vi "Mcp2210 Write EE Prom.vi"(8 "error in (no error)":errorcluster, 9 "value":u8, 10 "address":u8, 11 "handle":i32) -> (0 "error out":errorcluster, 3 "handle out":i32)   [LabVIEW 2015, in "mcp2210.lvlib"]
doc: "Write one byte at the EEPROM memory address provided as parameter.\nThe EEPROM size is 256 bytes.\nThe function returns negative error code in case of failure.\nIf the error code is \"M_E_ERR_BLOCKED_ACCESS\" the write failure is due to the device being either\npassword protected or permanently locked. M_Mcp2210_GetAccessStatus() API provides the details about\ndevice protection status. If the device is not permanently locked, the password protection can be\nunlocked or disabled by using the access control API.\nParameters:\nInputs:\n- IntPtr handle - The USB device handle. Cannot be NULL.\n- unsigned char address - the EEPROM location to write to.\n- unsigned char content - the value to store at the EEPROM address.\nOutputs:\n- none\nReturns:\n- 0 for success: M_E_SUCCESS\n- negative error code: M_E_ERR_NULL, M_E_ERR_INVALID_HANDLE_VALUE\nM_E_ERR_HID_TIMEOUT, M_E_ERR_HID_RW_FILEIO, M_E_ERR_UNKOWN_ERROR\nM_E_ERR_CMD_ECHO, M_E_ERR_CMD_FAILED\nM_E_ERR_BLOCKED_ACCESS\n\nMCP2210_DLL_UM_API int __stdcall Mcp2210_WriteEEProm(void *handle, unsigned char address, unsigned char content);"
uses:
  <userlib>/mcp2210/mcp2210.lvlib
  <userlib>/mcp2210/mcp2210_dll_um_x86.dll
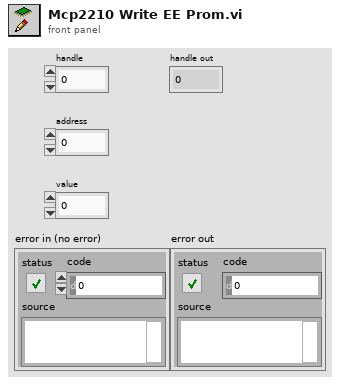
[diagram p1: front panel]
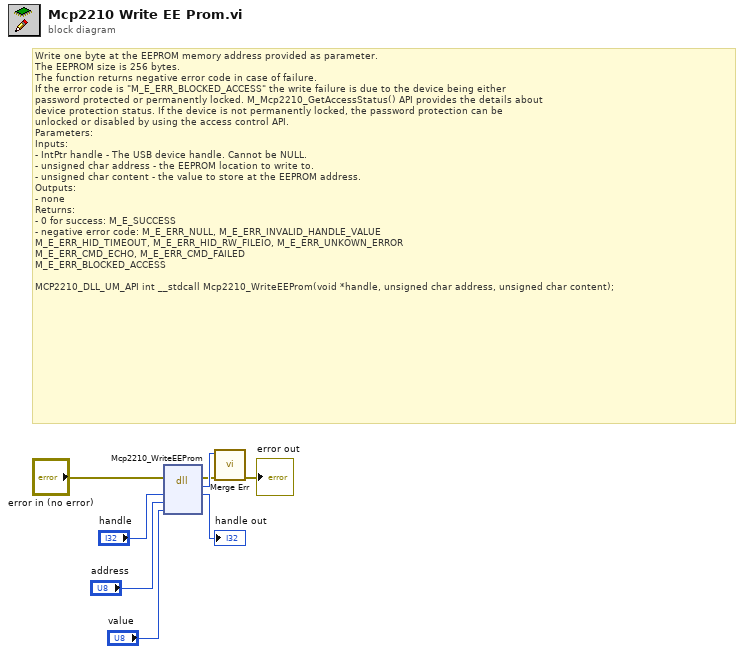
[diagram p0: block diagram]
diagram:
  # "Write one byte at the EEPROM memory address provided as parameter.\nThe EEPROM size is 256 bytes.\nThe function returns negative error code in case of failure.\nIf the error code is \"M_E_ERR_BLOCKED_ACCESS\" the write failure is due to the device being either\npassword protected or permanently locked. M_Mcp2210_GetAccessStatus() API provides the details about\ndevice protection status. If the device is not permanently locked, the password protection can be\nunlocked or disabled by using the access control API.\nParameters:\nInputs:\n- IntPtr handle - The USB device handle. Cannot be NULL.\n- unsigned char address - the EEPROM location to write to.\n- unsigned char content - the value to store at the EEPROM address.\nOutputs:\n- none\nReturns:\n- 0 for success: M_E_SUCCESS\n- negative error code: M_E_ERR_NULL, M_E_ERR_INVALID_HANDLE_VALUE\nM_E_ERR_HID_TIMEOUT, M_E_ERR_HID_RW_FILEIO, M_E_ERR_UNKOWN_ERROR\nM_E_ERR_CMD_ECHO, M_E_ERR_CMD_FAILED\nM_E_ERR_BLOCKED_ACCESS\n\nMCP2210_DLL_UM_API int __stdcall Mcp2210_WriteEEProm(void *handle, unsigned char address, unsigned char content);"
  n1 = dll-call lib="D:/LabVIEW 2015/user.lib/mcp2210/mcp2210_dll_um_x86.*" fn="Mcp2210_WriteEEProm"(error in="error in (no error)", "handle"="handle", "address"="address", "content"="value") -> (error out=w3:errorcluster, "return type"=w4:i32, "handle"=→"handle out":i32)  [unwired: 4 in, 1 out]
  n2 = call <userlib>:"Merge Err.vi"("error in (no error)"=w3, "return type"=w4) -> ("error out"=→"error out":errorcluster)  [unwired: 9 in]
